vi "字符串的使用.vi"() -> ()   [LabVIEW 2018]
panel:
  out "匹配后偏移量":i32
  out "子字符串之后":string
  out "匹配子字符串":string
  out "子字符串之前":string
  in  "偏移量(0) 2":i32
  in  "正则表达式":string
  in  "字符串":string
  out "替换后偏移量":i32
  out "替换数量":i32
  out "结果字符串":string
  in  "偏移量(0)":i32
  in  "替换字符串(\"\")":string
  in  "搜索字符串":string
  in  "忽略大小写？(F)":bool
  in  "替换全部？(F)":bool
  in  "输入字符串":string
  out "长度":i32
  in  "计算长度":string
  out "数值 2":dbl
  in  "数值":dbl
  out "布尔 2":bool
  in  "布尔":bool
  out "组合框输出":string
  in  "组合框":string(combo)
  out "输出":string
  in  "输入":string
  # "组合框的使用"
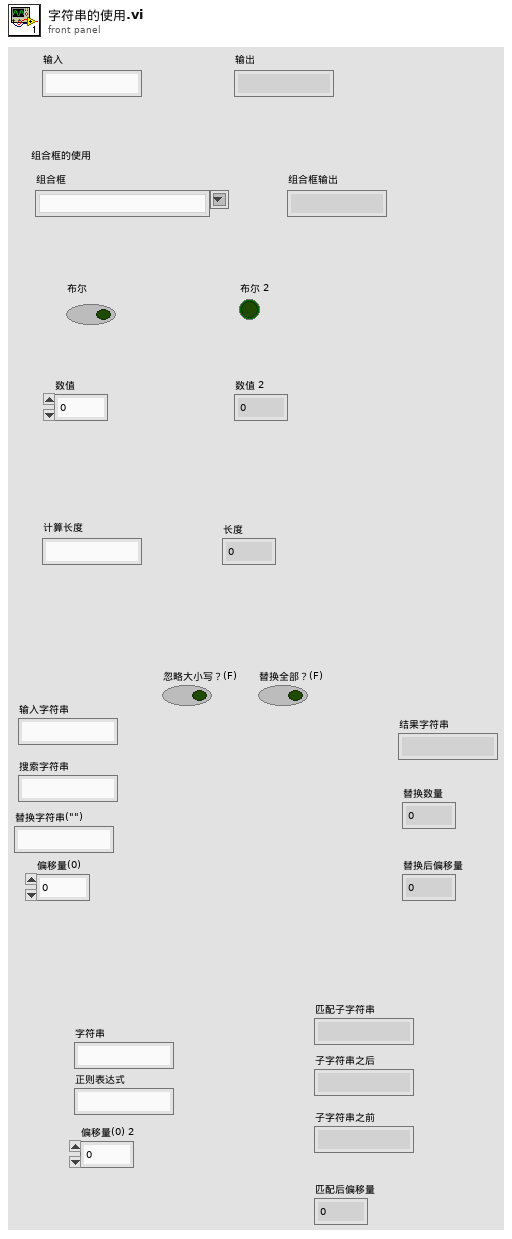
[diagram p1: front panel]
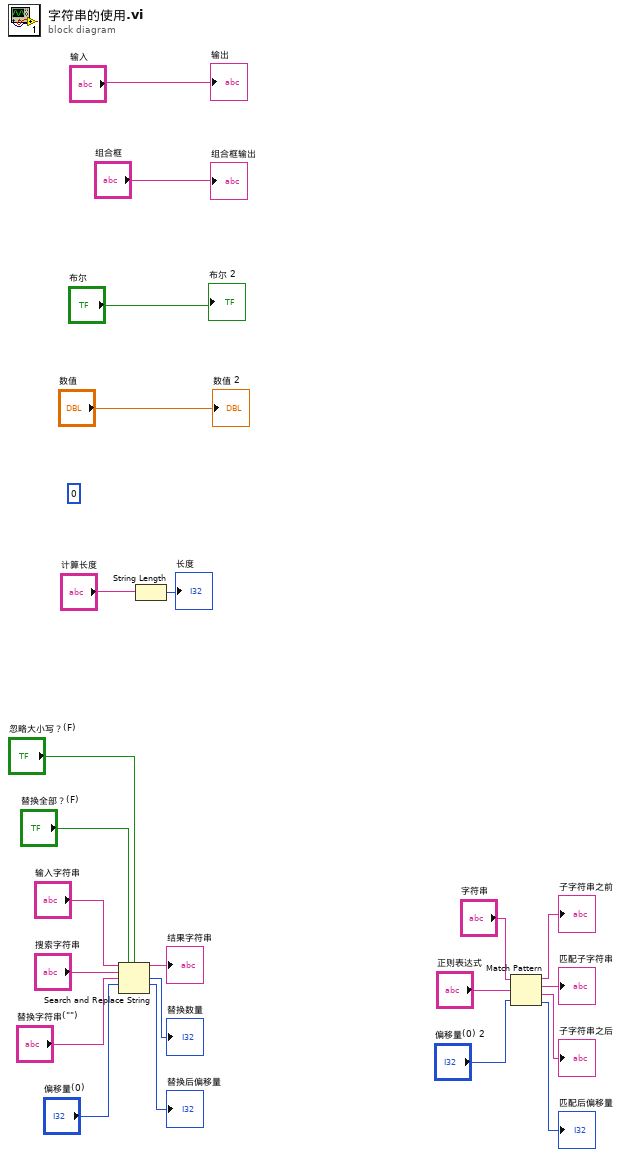
[diagram p0: block diagram]
diagram:
  (unwired) 0
  n1 = Search and Replace String(replace all?="替换全部？(F)", case sensitive?="忽略大小写？(F)", input string="输入字符串", search string="搜索字符串", replace string="替换字符串(\"\")", offset="偏移量(0)") -> (result string=→"结果字符串":string, number of replacements=→"替换数量":i32, offset past replacement=→"替换后偏移量":i32)  [unwired: 2 in, 1 out]
  n2 = String Length(string="计算长度") -> (length=→"长度":i32)
  n3 = Match Pattern(string="字符串", regular expression="正则表达式", offset (0)="偏移量(0) 2") -> (before substring=→"子字符串之前":string, match substring=→"匹配子字符串":string, after substring=→"子字符串之后":string, offset past match=→"匹配后偏移量":i32)
  "输出" <- "输入"
  "组合框输出" <- "组合框"
  "布尔 2" <- "布尔"
  "数值 2" <- "数值"
